vi "append_to_log.vi"(8 "error in":errorcluster, 11 "string":string) -> (0 "error out":errorcluster)   [LabVIEW 2014]
uses:
  Globals.vi
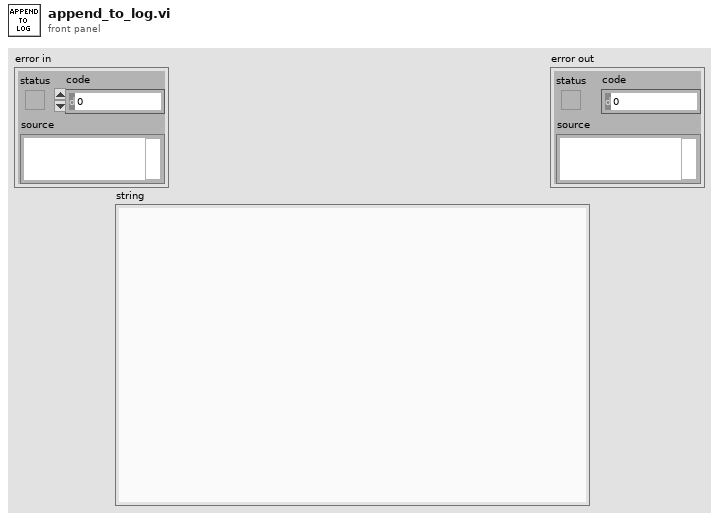
[diagram p1: front panel]
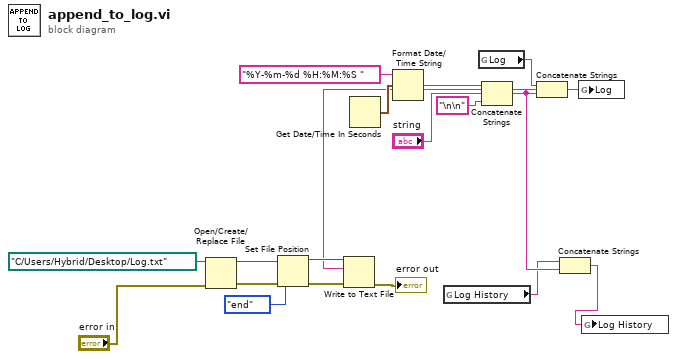
[diagram p0: block diagram]
diagram:
  n1 = Open/Create/Replace File(file path (use dialog)=path "C:/Users/Hybrid/Desktop/Log.txt", error in="error in") -> (refnum out=w9:refnum<file>, error out=w7:errorcluster)  [unwired: 4 in, 1 out]
  n2 = Set File Position(refnum=w9, from (0:start)=enum16{"start", "end", "current"}."end", error in=w7) -> (refnum out=w8:refnum<file>, error out=w6:errorcluster)  [unwired: 1 in]
  n3 = Get Date/Time In Seconds() -> (seconds since 1Jan1904=w18:timestamp)
  n4 = Format Date/Time String(time format string (%c)="%Y-%m-%d %H:%M:%S ", seconds (now)=w18) -> (date/time string=w16:string)  [unwired: 1 in]
  n5 = global read "Globals.vi" "Log History"() -> (w11:string)
  n6 = global read "Globals.vi" "Log"() -> (w13:string)
  n7 = Concatenate Strings(w16, "string", "\n\n" ("string")) -> (w12:string)
  n8 = Concatenate Strings(w13, w12) -> (w4:string)
  n9 = Write to Text File(file (use dialog)=w8, text=w4, error in=w6) -> (error out=→"error out":errorcluster)  [unwired: 1 in, 2 out]
  n10 = Concatenate Strings(w11, w12) -> (w10:string)
  n11 = global write "Globals.vi" "Log"(w4) -> ()
  n12 = global write "Globals.vi" "Log History"(w10) -> ()
